vi "log initial config.vi"(8 "error in (no error)":errorcluster, 11 "Socket in":refnum<class "Socket.lvclass">) -> (0 "error out":errorcluster, 3 "Socket out":refnum<class "Socket.lvclass">)   [LabVIEW 2018, in "Socket.lvclass"]
uses:
  Socket.lvclass
  <vilib>/addons/zeromq/socket_type.ctl
  <vilib>/addons/zeromq/socket_options.ctl
  Socket.lvclass/Socket.ctl
  Log File/CM_Log File.lvclass
  <vilib>/addons/zeromq/zeromq.lvlib
panel:
  out "Name":string
  out "ID":u32
  out "option":T1=enum."ZMQ_SWAP"
  out "IP":string="tcp://"
  out "linger (ms)":i32
  out "socket type":T2
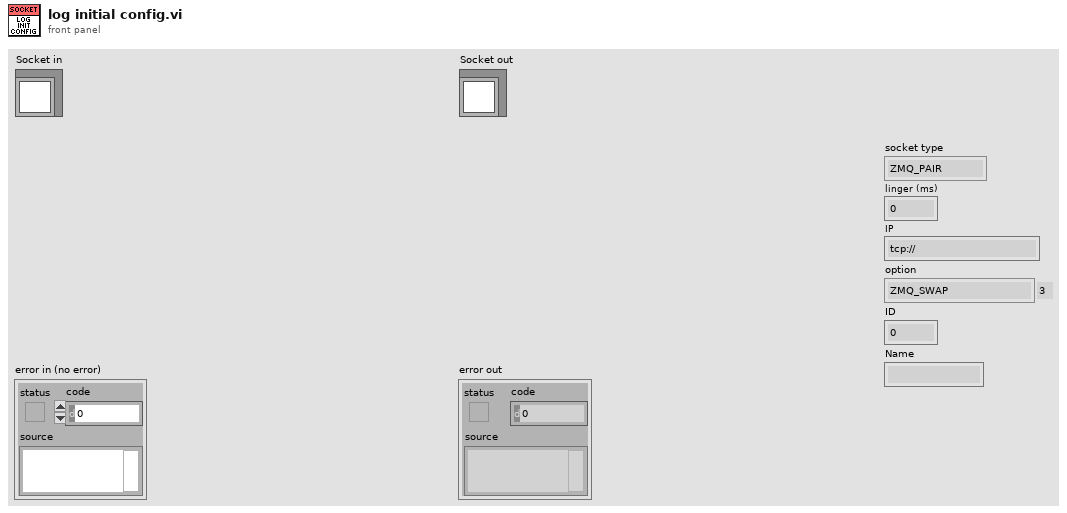
[diagram p1: front panel]
types:
  T1 = typedef "zeromq.lvlib/socket_options.ctl" = enum8{"NONE", "ZMQ_HWM", "<2>", "ZMQ_SWAP", "ZMQ_AFFINITY", "ZMQ_ROUTING_ID", "ZMQ_SUBSCRIBE", "ZMQ_UNSUBSCRIBE", "ZMQ_RATE", "ZMQ_RECOVERY_IVL", "ZMQ_MCAST_LOOP", "ZMQ_SNDBUF", "ZMQ_RCVBUF", "ZMQ_RCVMORE", "ZMQ_FD", "ZMQ_EVENTS", "ZMQ_TYPE", "ZMQ_LINGER", "ZMQ_RECONNECT_IVL", "ZMQ_BACKLOG", "ZMQ_RECOVERY_IVL_MSEC", "ZMQ_RECONNECT_IVL_MAX", "ZMQ_MAXMSGSIZE", "ZMQ_SNDHWM", "ZMQ_RCVHWM", "ZMQ_MULTICAST_HOPS", "<26>", "ZMQ_RCVTIMEO", "ZMQ_SNDTIMEO", "<29>", "<30>", "ZMQ_IPV4ONLY", "ZMQ_LAST_ENDPOINT", "ZMQ_ROUTER_MANDATORY", "ZMQ_TCP_KEEPALIVE", "ZMQ_TCP_KEEPALIVE_CNT", "ZMQ_TCP_KEEPALIVE_IDLE", "ZMQ_TCP_KEEPALIVE_INTVL", "ZMQ_TCP_ACCEPT_FILTER", "ZMQ_IMMEDIATE", "ZMQ_XPUB_VERBOSE", "ZMQ_ROUTER_RAW", "ZMQ_IPV6", "ZMQ_MECHANISM", "ZMQ_PLAIN_SERVER", "ZMQ_PLAIN_USERNAME", "ZMQ_PLAIN_PASSWORD", "ZMQ_CURVE_SERVER", "ZMQ_CURVE_PUBLICKEY", "ZMQ_CURVE_SECRETKEY", "ZMQ_CURVE_SERVERKEY", "ZMQ_PROBE_ROUTER", "ZMQ_REQ_CORRELATE", "ZMQ_REQ_RELAXED", "ZMQ_CONFLATE", "ZMQ_ZAP_DOMAIN", "ZMQ_ROUTER_HANDOVER", "ZMQ_TOS", "ZMQ_IPC_FILTER_PID", "ZMQ_IPC_FILTER_UID", "ZMQ_IPC_FILTER_GID", "ZMQ_CONNECT_ROUTING_ID", "ZMQ_GSSAPI_SERVER", "ZMQ_GSSAPI_PRINCIPAL", "ZMQ_GSSAPI_SERVICE_PRINCIPAL", "ZMQ_GSSAPI_PLAINTEXT", "ZMQ_HANDSHAKE_IVL", "<67>", "ZMQ_SOCKS_PROXY", "ZMQ_XPUB_NODROP", "ZMQ_BLOCKY", "ZMQ_XPUB_MANUAL", "ZMQ_XPUB_WELCOME_MSG", "ZMQ_STREAM_NOTIFY", "ZMQ_INVERT_MATCHING", "ZMQ_HEARTBEAT_IVL", "ZMQ_HEARTBEAT_TTL", "ZMQ_HEARTBEAT_TIMEOUT", "ZMQ_XPUB_VERBOSER", "ZMQ_CONNECT_TIMEOUT", "ZMQ_TCP_MAXRT", "ZMQ_THREAD_SAFE", "<82>", "<83>", "ZMQ_MULTICAST_MAXTPDU", "ZMQ_VMCI_BUFFER_SIZE", "ZMQ_VMCI_BUFFER_MIN_SIZE", "ZMQ_VMCI_BUFFER_MAX_SIZE", "ZMQ_VMCI_CONNECT_TIMEOUT", "ZMQ_USE_FD", "ZMQ_GSSAPI_PRINCIPAL_NAMETYPE", "ZMQ_GSSAPI_SERVICE_PRINCIPAL_NAMETYPE", "ZMQ_BINDTODEVICE", "ZMQ_ZAP_ENFORCE_DOMAIN", "ZMQ_LOOPBACK_FASTPATH", "ZMQ_METADATA", "ZMQ_MULTICAST_LOOP", "ZMQ_ROUTER_NOTIFY"}
  T2 = typedef "zeromq.lvlib/socket_type.ctl" = enum8{"ZMQ_PAIR", "ZMQ_PUB", "ZMQ_SUB", "ZMQ_REQ", "ZMQ_REP", "ZMQ_DEALER", "ZMQ_ROUTER", "ZMQ_PULL", "ZMQ_PUSH", "ZMQ_XPUB", "ZMQ_XSUB", "ZMQ_STREAM", "ZMQ_SERVER", "ZMQ_CLIENT", "ZMQ_RADIO", "ZMQ_DISH", "ZMQ_GATHER", "ZMQ_SCATTER", "ZMQ_DGRAM"}
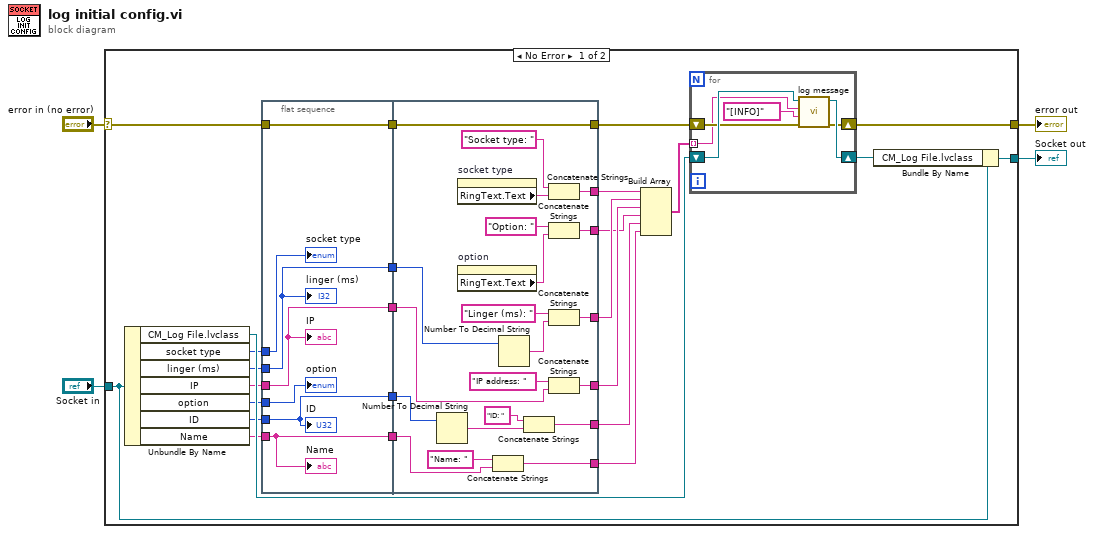
[diagram p0: block diagram]
diagram:
  n1 = case shown="No Error" "error in (no error)" {
    selector: "error in (no error)" -> [w24 w65]
    tunnel: [w29 w65] -> w3
    tunnel: [w26 w64] -> w1
    tunnel: "Socket in" -> [w27 w64]
    frame No Error {
      n2 = Unbundle By Name(w27) -> ("CM_Log File.lvclass"=w28:refnum<class "CM_Log File.lvclass">, "socket type"=w23:T2, "linger (ms)"=w21:i32, "IP"=w22:string, "option"=w20:T1, "ID"=w19:u32, "Name"=w18:string)
      n3 = flat-sequence {
        tunnel: w24 -> [w36]
        tunnel: w23 -> [w35]
        tunnel: w22 -> [w33]
        tunnel: w21 -> [w32]
        tunnel: w20 -> [w34]
        tunnel: w19 -> [w30]
        tunnel: w18 -> [w31]
        tunnel: [w36] -> w16
        tunnel: [w33] -> w15
        tunnel: [w32] -> w14
        tunnel: [w31] -> w13
        tunnel: [w30] -> w12
        tunnel: [w57] -> w17
        tunnel: w16 -> [w57]
        tunnel: w15 -> [w53]
        tunnel: w14 -> [w51]
        tunnel: w13 -> [w47]
        tunnel: w12 -> [w46]
        tunnel: [w42] -> w11
        tunnel: [w41] -> w10
        tunnel: [w40] -> w9
        tunnel: [w39] -> w8
        tunnel: [w38] -> w7
        tunnel: [w37] -> w6
        frame #0 {
          "socket type" <- w35
          "IP" <- w33
          "linger (ms)" <- w32
          "option" <- w34
          "ID" <- w30
          "Name" <- w31
        }
        frame #1 {
          n4 = Number To Decimal String(number=w46) -> (decimal integer string=w45:string)  [unwired: 1 in]
          n5 = property on="socket type" class="Enum (strict)"() -> ("RingText.Text"=w56:string)  [unwired: 2 in, 2 out]
          n6 = property on="option" class="Enum (strict)"() -> ("RingText.Text"=w43:string)  [unwired: 2 in, 2 out]
          n7 = Concatenate Strings("Name: " ("string"), w47) -> (w37:string)
          n8 = Number To Decimal String(number=w51) -> (decimal integer string=w50:string)  [unwired: 1 in]
          n9 = Concatenate Strings("ID: " ("string"), w45) -> (w38:string)
          n10 = Concatenate Strings("Socket type: " ("string"), w56) -> (w42:string)
          n11 = Concatenate Strings("Option: " ("string"), w43) -> (w39:string)
          n12 = Concatenate Strings("Linger (ms): " ("string"), w50) -> (w41:string)
          n13 = Concatenate Strings("IP address: " ("string"), w53) -> (w40:string)
        }
      }
      n14 = Build Array(w11, w10, w9, w8, w7, w6) -> (w5:string[])
      n15 = for {
        shift-right: [w59] -> w29
        shift-left: w17 -> [w60]
        shift-right: [w61] -> w25
        shift-left: w28 -> [w62]
        tunnel: w5 -> [w58] mode=indexing
        n16 = call-dynamic "log message.vi"("error in (no error)"=w60, "message type"="[INFO]", "Message to log"=w58, "Log File in"=w62) -> ("error out"=w59:errorcluster, "Log File out"=w61:refnum<class "CM_Log File.lvclass">)  [unwired: 6 in]
      }
      n17 = Bundle By Name(cluster=w27, "CM_Log File.lvclass"=w25) -> (w26:refnum<class "Socket.lvclass">)
    }
    frame Error {
    }
  }
  "error out" <- w3
  "Socket out" <- w1
